vi "Validate CSRF Token.vi"(8 "error in (no error)":errorcluster, 9 "Token":string, 10 "Token ID":string, 11 "Session In":refnum<class "Session.lvclass">) -> (0 "error out":errorcluster, 3 "Session":refnum<class "Session.lvclass">)   [LabVIEW 2020, in "HTTP Server.lvlib"]
uses:
  HTTP Server.lvlib
  Session/Session.lvclass
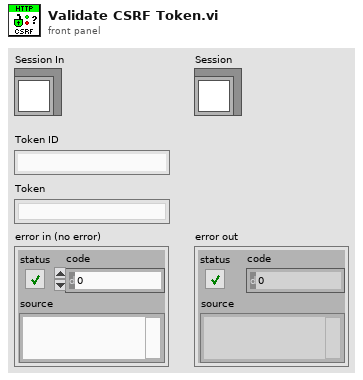
[diagram p1: front panel]
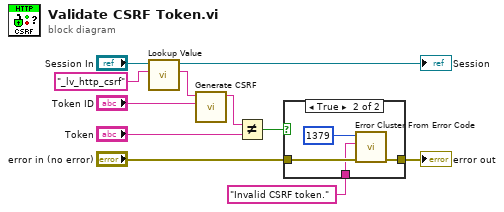
[diagram p0: block diagram]
diagram:
  n1 = call "Lookup Value.vi"("Name"="_lv_http_csrf", "Session in"="Session In") -> ("Value"=w9:string, "Session out"=→"Session":refnum<class "Session.lvclass">)  [unwired: 6 in, 2 out]
  n2 = call "Generate CSRF.vi"("Token ID"="Token ID", "Key"=w9) -> ("Generated Token"=w6:string)  [unwired: 9 in]
  n3 = Not Equal?(x=w6, y="Token") -> (x != y?=w4:bool)
  n4 = case shown="True" w4 {
    tunnel: "error in (no error)" -> [w12 w15]
    tunnel: [w12 w14] -> w2
    tunnel: "Invalid CSRF token." -> [_ w13]
    frame False {
    }
    frame True {
      n5 = call <vilib>:"Error Cluster From Error Code.vi"("error in (no error)"=w15, "error message (\"\")"=w13, "error code (0)"=1379) -> ("error out"=w14:errorcluster)  [unwired: 6 in]
    }
  }
  "error out" <- w2
